vi "Message type that caused error.vi"(11 "IErrorHandler in":refnum<class "IErrorHandler.lvclass">) -> (2 "Error in response to message type":T1, 3 "IErrorHandler out":refnum<class "IErrorHandler.lvclass">)   [LabVIEW 2020, in "wamplv.lvlib" / "IErrorHandler.lvclass"]
uses:
  IErrorHandler.lvclass
  TypeDefs/WAMP Message Codes.ctl
  wamplv.lvlib
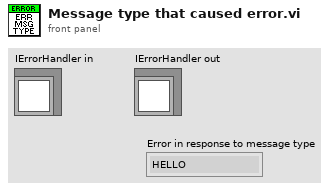
[diagram p1: front panel]
types:
  T1 = typedef "wamplv.lvlib/WAMP Message Codes.ctl" = enum8{"HELLO", "WELCOME", "CHALLENGE", "AUTHENTICATE", "ABORT", "GOODBYE", "ERROR", "PUBLISH", "PUBLISHED", "SUBSCRIBE", "SUBSCRIBED", "UNSUBSCRIBE", "UNSUBSCRIBED", "EVENT", "CALL", "RESULT", "REGISTER", "REGISTERED", "UNREGISTER", "UNREGISTERED", "INVOCATION", "YIELD"}
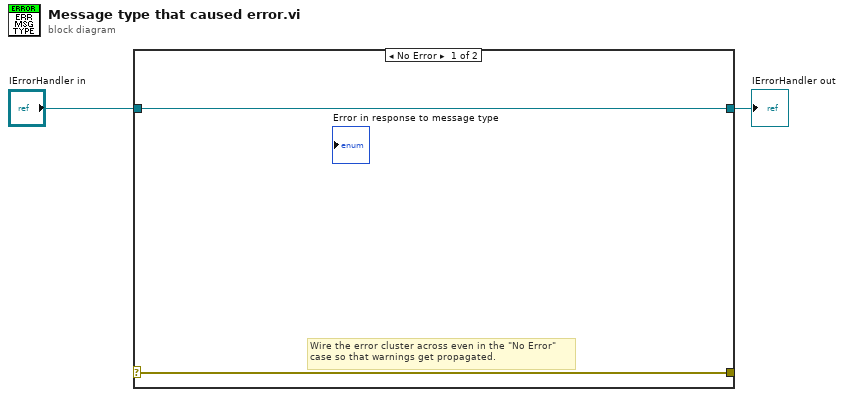
[diagram p0: block diagram]
diagram:
  n1 = case shown="No Error" {
    selector: _ -> [w3 w6]
    tunnel: [w3 w6] -> _
    tunnel: [w4 w5] -> w1
    tunnel: "IErrorHandler in" -> [w4 w5]
    frame No Error {
      # "Wire the error cluster across even in the \"No Error\"\ncase so that warnings get propagated."
    }
    frame Error {
    }
  }
  "IErrorHandler out" <- w1
